vi "Hatch Piston TeleOp.vi"(11 "Cluster":cluster{"Cluster":T1}) -> ()   [LabVIEW 2018]
uses:
  Controller Values.ctl
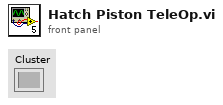
[diagram p1: front panel]
types:
  T1 = typedef "Controller Values.ctl" = cluster{"Left Joystick Axes ":dbl[], "Right Joystick Axes":dbl[], "Left Joystick Buttons":bool[], "Right Joystick Buttons":bool[], "DDR Buttons":bool[], "XBox Axes":dbl[], "XBox Buttons":bool[], "XBox POVs":i16[]}
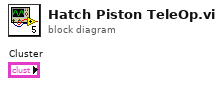
[diagram p0: block diagram]
diagram:
